vi "GetSetFloat.vi"(7 "Set?":bool, 8 "error in (no error)":errorcluster, 9 "Value In":dbl, 10 "Name":string, 11 "Camera in":refnum<class "Camera.lvclass">) -> (0 "error out":errorcluster, 1 "Value Out":dbl)   [LabVIEW 2020, in "Camera.lvclass"]
uses:
  Camera.lvclass
  Camera.lvclass/Camera.ctl
  bin/gindustrialcam_32-1.dll
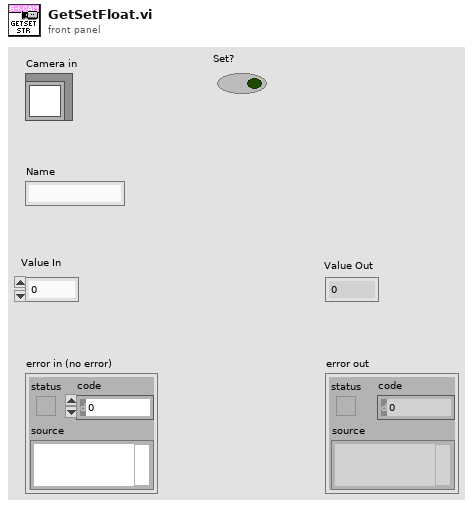
[diagram p1: front panel]
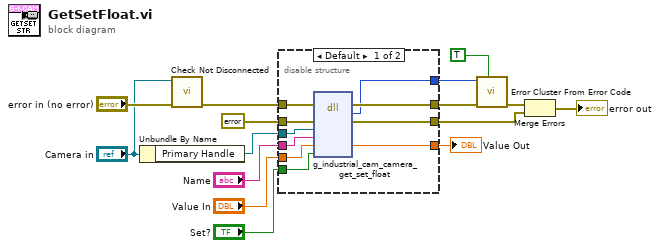
[diagram p0: block diagram]
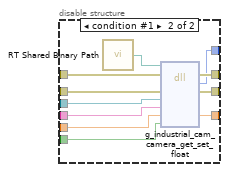
[diagram p2: hidden frame]
diagram:
  n1 = Unbundle By Name("Camera in") -> ("Primary Handle"=w5:refnum<data-value>)
  n2 = call "Check Not Disconnected.vi"("error in (no error)"="error in (no error)", "Camera in"="Camera in") -> ("error out"=w2:errorcluster)  [unwired: 9 in]
  n3 = disable-structure shown="Default" {
    disable-tunnel: [w25 w36] -> w15
    disable-tunnel: [w24 w35] -> w14
    disable-tunnel: [w23 w34] -> w12
    disable-tunnel: errorcluster {"status"=FALSE, "code"=0, "source"=""} ("error constant") -> [w22 w33]
    disable-tunnel: "Name" -> [w21 w32]
    disable-tunnel: "Set?" -> [w20 w31]
    disable-tunnel: w5 -> [w19 w30]
    disable-tunnel: "Value In" -> [w18 w29]
    disable-tunnel: [w17 w28] -> w3
    disable-tunnel: w2 -> [w16 w27]
    frame condition #0 (active) {
      n4 = dll-call lib="C:/serenial/lib/g-industrial-camera/LabVIEW/g_industrial_cam/bin/gindustrialcam_*-1.*" fn="g_industrial_cam_camera_get_set_float"(error in=w16, "err"=w22, "edvr"=w19, "name"=w21, "value"=w18, "set"=w20) -> (error out=w25:errorcluster, "Mg_Error"=w24:i32, "err"=w23:errorcluster, "value"=w17:dbl)  [unwired: 5 in, 1 out]
    }
    frame condition #1 {
      n5 = call "RT Shared Binary Path.vi"() -> ("Path"=w26:path)
      n6 = dll-call lib="C:/serenial/lib/g-industrial-camera/LabVIEW/g_industrial_cam/bin/gindustrialcam_*-1.*" fn="g_industrial_cam_camera_get_set_float"(path in=w26, error in=w27, "err"=w33, "edvr"=w30, "name"=w32, "value"=w29, "set"=w31) -> (error out=w36:errorcluster, "Mg_Error"=w35:i32, "err"=w34:errorcluster, "value"=w28:dbl)  [unwired: 4 in, 1 out]
    }
  }
  "Value Out" <- w3
  n7 = call <vilib>:"Error Cluster From Error Code.vi"("show call chain? (False)"=TRUE, "error in (no error)"=w15, "error code (0)"=w14) -> ("error out"=w13:errorcluster)  [unwired: 6 in]
  n8 = Merge Errors(w13, w12) -> (→"error out":errorcluster)
